vi "Load PQ .bin File Information.vi"(8 "Error In":errorcluster, 11 "File Path":path) -> (0 "Error Out":errorcluster, 1 "Data Description":string, 3 "FLI Data File Information":T1, 4 "Load Time (s)":dbl)   [LabVIEW 2021, in "PicoQuant.lvlib"]
doc: "Uncheck the <B>Process</B> checkbox to read only the header (and fill the PicoQuant Data File Information structure).\n\nCheck the box to actually read and decode the data.\n\nThe <B>Max # Gates</B> control is used to set the level of nanotime binning (smaller is better in terms of memory usage).\n\nWhen the file is decoded (green LED), scroll to the right to show the <B>Stop</B> button and display controls used to represent the data in an Intensity Graph (Intensity Image or individual gate images) and represent individual pixel decays at the cursor location."
uses:
  PicoQuant.lvlib
  AlliGator/AlliGator FLI Data File Information.ctl
  Phasor/Phasor Fluorescence Lifetime Parameters v3.ctl
  AlliGator/AlliGator FLI Dataset Type.ctl
  Extended PQ .bin Dataset Information.ctl
  BIN File Information.ctl
  AlliGator/AlliGator Load Single Gate Image from .bin File.vi
  AlliGator/AlliGator HDF5.lvlib
  AlliGator/AlliGator Files.lvlib
  Phasor/Phasor.lvlib
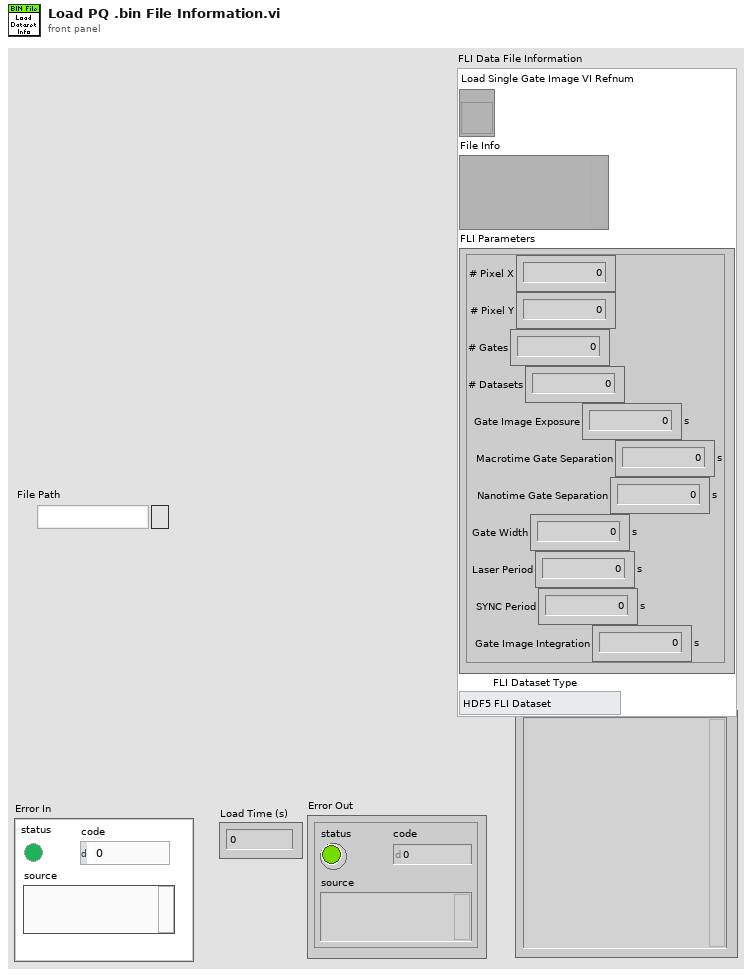
[diagram p1: front panel]
types:
  T1 = typedef "AlliGator HDF5.lvlib/AlliGator FLI Data File Information.ctl" = cluster{"Load Single Gate Image VI Refnum":refnum<vi>, "File Info":variant, "FLI Parameters":T2, "FLI Dataset Type":T3}
  T2 = typedef "Phasor.lvlib/Phasor Fluorescence Lifetime Parameters v3.ctl" = cluster{"# Pixel X":i32, "# Pixel Y":i32, "# Gates":i32, "# Datasets":i32, "Gate Image Exposure":dbl[unit], "Macrotime Gate Separation":dbl[unit], "Nanotime Gate Separation":dbl[unit], "Gate Width":dbl[unit], "Laser Period":dbl[unit], "SYNC Period":dbl[unit], "Gate Image Integration":dbl[unit]}
  T3 = typedef "AlliGator Files.lvlib/AlliGator FLI Dataset Type.ctl" = enum16{"HDF5 FLI Dataset", "Gate Image Folder", ".sdt FLI Dataset (Becker & Hickl)", ".ptu FLI Dataset (PicoQuant)", "SS1 FLI Dataset", "SS2 FLI Dataset", "I/m/phi Dataset", ".bin FLI Dataset (PicoQuant Binned)", ".bin FLI Dataset (Piccolo Binned)"}
  T4 = typedef "PicoQuant.lvlib/Extended PQ .bin Dataset Information.ctl" = cluster{"File Path":path, "offset (in bytes)":i64, "BIN dataset Information":T5}
  T5 = typedef "PicoQuant.lvlib/BIN File Information.ctl" = cluster{"# Pixels X":i32, "# Pixels Y":i32, "Spatial Resolution":dbl[unit], "# TCSPC Bins":i32, "Temporal Resolution":dbl[unit]}
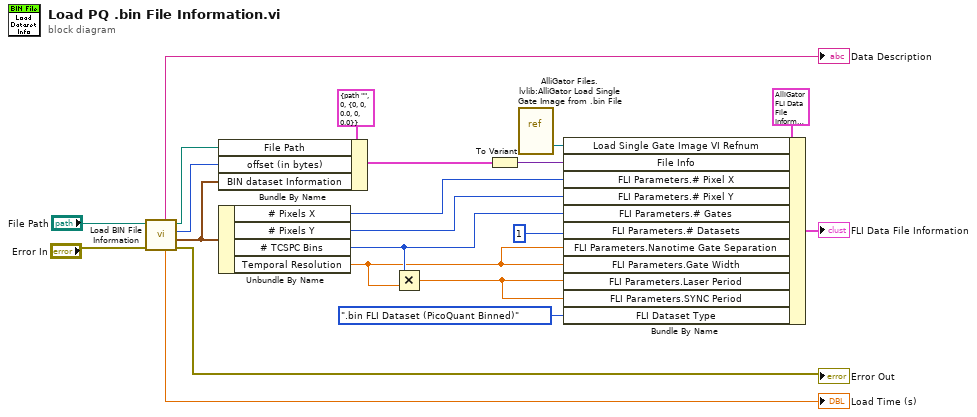
[diagram p0: block diagram]
diagram:
  n1 = call "Load BIN File Information.vi"("error in (no error)"="Error In", "File Path"="File Path") -> ("error out"=→"Error Out":errorcluster, "BIN dataset Information"=w5:T5, "offset (in bytes)"=w3:i64, "File Path out"=w4:path, "CPU (s)"=→"Load Time (s)":dbl, "Data Description"=→"Data Description":string)  [unwired: 4 in]
  n2 = Bundle By Name(cluster=T4 {"File Path"=path "", "offset (in bytes)"=0, "BIN dataset Information"={"# Pixels X"=0, "# Pixels Y"=0, "Spatial Resolution"=0.0, "# TCSPC Bins"=0, "Temporal Resolution"=0.0}} ("output cluster"), "File Path"=w4, "offset (in bytes)"=w3, "BIN dataset Information"=w5) -> (w1:T4)
  n3 = Unbundle By Name(w5) -> ("# Pixels X"=w10:i32, "# Pixels Y"=w9:i32, "# TCSPC Bins"=w8:i32, "Temporal Resolution"=w7:dbl[unit])
  n4 = Multiply(x=w8, y=w7) -> (x*y=w6:dbl[unit])
  n5 = To Variant(anything=w1) -> (Variant=w20:variant)
  n6 = vi-ref "AlliGator Files.lvlib:AlliGator Load Single Gate Image from .bin File.vi"() -> (w17:refnum<vi>)
  n7 = Bundle By Name(cluster=T1 {"Load Single Gate Image VI Refnum"=refnum, "File Info"=variant, "FLI Parameters"={"# Pixel X"=0, "# Pixel Y"=0, "# Gates"=0, "# Datasets"=0, "Gate Image Exposure"=0.0, "Macrotime Gate Separation"=0.0, "Nanotime Gate Separation"=0.0, "Gate Width"=0.0, "Laser Period"=0.0, "SYNC Period"=0.0, "Gate Image Integration"=0.0}, "FLI Dataset Type"=enum."HDF5 FLI Dataset"} ("FLI Data File Information"), "Load Single Gate Image VI Refnum"=w17, "File Info"=w20, "FLI Parameters.# Pixel X"=w10, "FLI Parameters.# Pixel Y"=w9, "FLI Parameters.# Gates"=w8, "FLI Parameters.# Datasets"=1, "FLI Parameters.Nanotime Gate Separation"=w7, "FLI Parameters.Gate Width"=w7, "FLI Parameters.Laser Period"=w6, "FLI Parameters.SYNC Period"=w6, "FLI Dataset Type"=AlliGator_FLI_Dataset_Type.".bin FLI Dataset (PicoQuant Binned)") -> (→"FLI Data File Information":T1)
